vi "Read Limit Volt.vi"(8 "error in":errorcluster, 11 "PowerSupply in":refnum<class "PowerSupply.lvclass">) -> (0 "error out":errorcluster, 2 "OverVolt_Protect":dbl, 3 "PowerSupply out":refnum<class "PowerSupply.lvclass">)   [LabVIEW 2019, in "PowerSupply.lvlib" / "PowerSupply.lvclass"]
uses:
  Library/PowerSupply.lvclass
  Library/PowerSupply.lvclass/PowerSupply.ctl
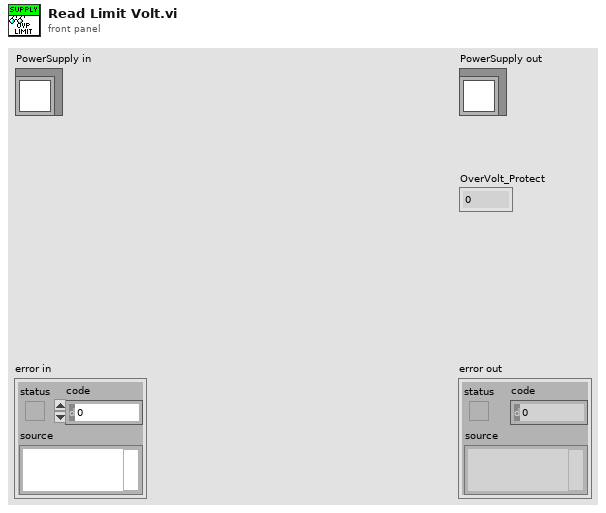
[diagram p1: front panel]
types:
  T1 = typedef "PowerSupply.lvlib/PowerSupply.lvclass/Settings.ctl" = cluster{"Voltage":dbl, "Current":dbl, "Output":bool, "OverVolt_Protect":dbl, "OverCurrent_Protect":dbl, "OVP":bool, "OCP":bool, "Interlock":bool, "Volt_Ramp":dbl, "Current_Ramp":dbl, "Sense Point":T2, "OCP Mode":T3}
  T2 = typedef "PowerSupply.lvlib/PowerSupply.lvclass/Sense Point.ctl" = enum16{"Local", "Remote"}
  T3 = typedef "PowerSupply.lvlib/PowerSupply.lvclass/OCP Mode.ctl" = enum16{"Shutdown", "Foldback"}
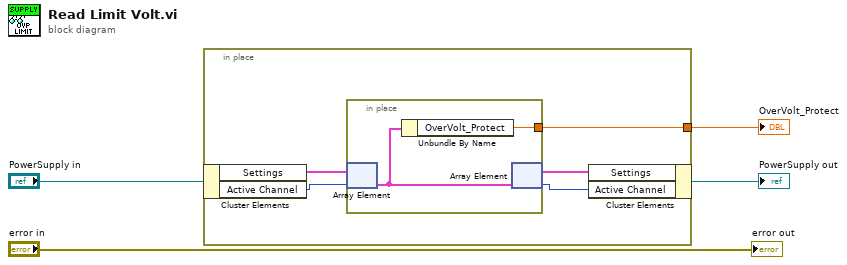
[diagram p0: block diagram]
diagram:
  n1 = in-place {
    in-place-border: [w9] -> w4
    n2 = in-place-cluster #1("PowerSupply in") -> ("Settings"=w8:T1[], "Active Channel"=w7:u32)
    n3 = in-place {
      in-place-border: [w10] -> w9
      n4 = in-place-array #2(w8, w7) -> (w11:T1)
      n5 = Unbundle By Name(w11) -> ("OverVolt_Protect"=w10:dbl)
      n6 = in-place-array #2(w11) -> (w6:T1[], w5:i32)
    }
    n7 = in-place-cluster #1("Settings"=w6, "Active Channel"=w5) -> (→"PowerSupply out":refnum<class "PowerSupply.lvclass">)
  }
  "OverVolt_Protect" <- w4
  "error out" <- "error in"
